vi "SubSystems.vi"(8 "error in":errorcluster) -> ()   [LabVIEW 2019]
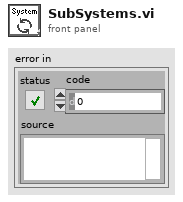
[diagram p1: front panel]
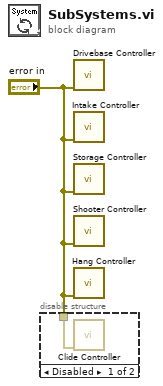
[diagram p0: block diagram]
diagram:
  n1 = disable-structure shown="Disabled" {
    disable-tunnel: "error in" -> [w2 _]
    frame Disabled {
      n2 = call "Clide Controller.vi"("error in"=w2) -> ()  [unwired: 11 in]
    }
    frame Enabled {
    }
  }
  n3 = call "Drivebase Controller.vi"("error in"="error in") -> ()  [unwired: 11 in]
  n4 = call "Intake Controller.vi"("error in"="error in") -> ()  [unwired: 11 in]
  n5 = call "Storage Controller.vi"("error in"="error in") -> ()  [unwired: 11 in]
  n6 = call "Shooter Controller.vi"("error in"="error in") -> ()  [unwired: 11 in]
  n7 = call "Hang Controller.vi"("error in"="error in") -> ()  [unwired: 11 in]
